vi "BC Next Frame Check.vi"(8 "error in (no error)":errorcluster, 11 "Bus Controller in":refnum<class "Bus Controller.lvclass">) -> (0 "error out":errorcluster, 3 "Bus Controller out":refnum<class "Bus Controller.lvclass">)   [LabVIEW 2020, in "Unit Tests.lvlib" / "Bus Controller.lvclass"]
uses:
  Bus Controller.lvclass
  Bus Controller.lvclass/Bus Controller.ctl
  Frames & Messages/TypeDefs/BC Condition Codes.ctl
  Frames & Messages/TypeDefs/BC Op Codes - Verbose.ctl
  <vilib>/addons/_JKI Toolkits/Caraya/classes/Assert/Assert True.vi
  Dependencies/FPGA Interface/FPGA Interface.lvclass
  <vilib>/addons/_JKI Toolkits/Caraya/classes/Test/Test.lvclass
  BCI-1553 API.lvlib
  <vilib>/addons/_JKI Toolkits/Caraya/classes/Assert/Assert.lvclass
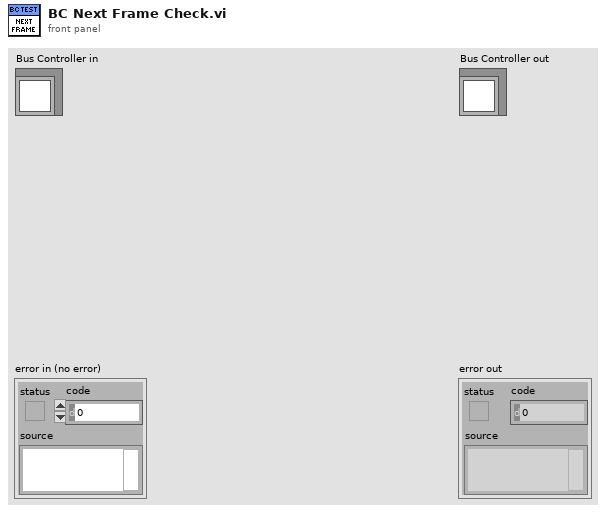
[diagram p1: front panel]
types:
  T1 = typedef "BCI-1553 API.lvlib/BC Op Codes - Verbose.ctl" = enum16{"EXECUTE MSG", "EXECUTE MSG GO", "JUMP", "CALL SUBROUTINE", "RETURN", "INTERRUPT REQUEST", "HALT", "DELAY", "WAIT FRAME TIMER = 0", "COMPARE FRAME TIMER", "COMPARE MSG TIMER", "LOAD TIME TAG CTR", "LOAD TIME TAG CTR HI", "LOAD FRAME TIMER", "START FRAME TIMER", "PUSH TIME TAG COUNT", "PUSH TIME TAG COUNT HI", "PUSH TIME TAG COUNT BOTH", "PUSH BLOCK STATUS WORD", "PUSH CURRENT VALUE", "PUSH INDIRECT", "WAIT EXT TRIGGER", "EXECUTE AND FLIP", "EXECUTE, FLIP, GO", "WRITE VALUE TO WMI", "WRITE VALUE TO MEM", "DECREMENT RAM, SKIP", "FLAG"}
  T2 = typedef "BCI-1553 API.lvlib/BC Condition Codes.ctl" = enum16{"GP0 == 1 || LT", "GP1 == 1 || NE", "GP2 == 1", "GP3 == 1", "GP4 == 1", "GP5 == 1", "GP6 == 1", "GP7 == 1", "NORESP", "FMTERR", "GOODBLOCK", "MSKSTATSET", "BADMSG", "1RETRY", "2RETRY", "ALWAYS"}
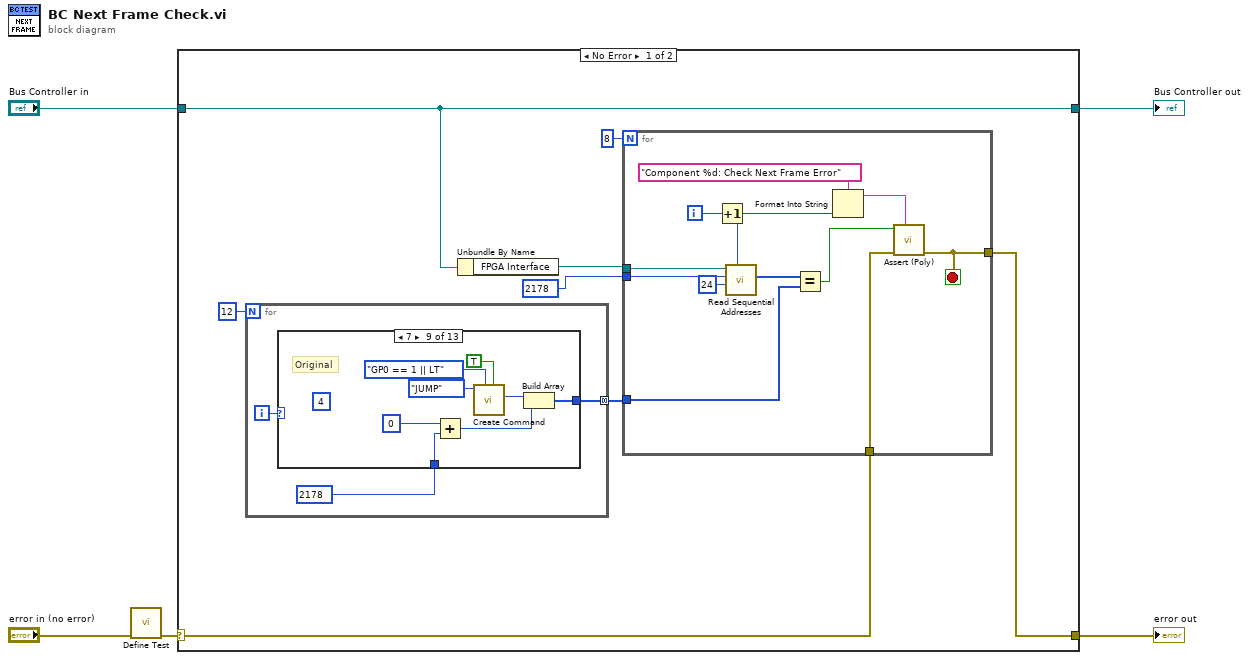
[diagram p0: block diagram]
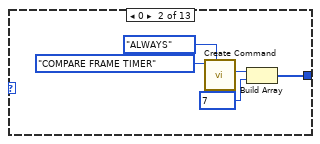
[diagram p3: hidden frame]
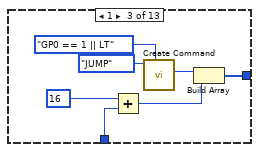
[diagram p4: hidden frame]
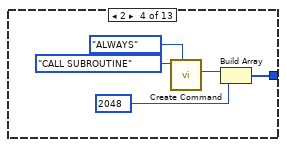
[diagram p5: hidden frame]
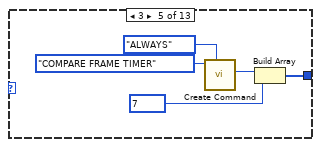
[diagram p6: hidden frame]
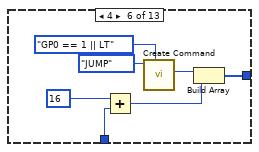
[diagram p7: hidden frame]
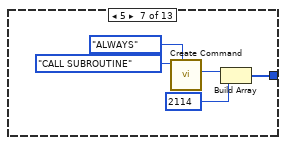
[diagram p8: hidden frame]
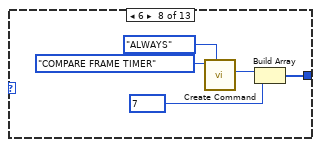
[diagram p9: hidden frame]
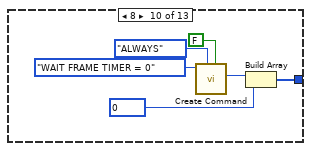
[diagram p10: hidden frame]
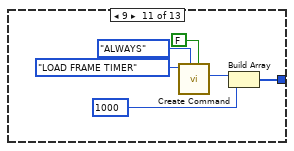
[diagram p11: hidden frame]
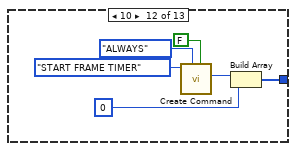
[diagram p12: hidden frame]
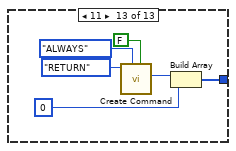
[diagram p13: hidden frame]
diagram:
  n1 = call <vilib>:"Define Test.vi"("error in (no error)"="error in (no error)") -> ("error out"=w1:errorcluster)  [unwired: 9 in, 1 out]
  n2 = case shown="No Error" w1 {
    selector: w1 -> [w8 w101]
    tunnel: [w7 w101] -> w5
    tunnel: [w11 w100] -> w3
    tunnel: "Bus Controller in" -> [w11 w100]
    frame No Error {
      n3 = for {
        N: 12 -> [_]
        tunnel: [w27] -> w12 mode=concatenating
        i -> [w28]
        n4 = case shown="7" w28 {
          tunnel: [_ w30 w37 w42 w47 w54 w59 w64 w72 w78 w84 w90 w96] -> w27
          tunnel: u16 2178 -> [_ _ w34 _ _ w51 _ _ w68 _ _ _ _]
          frame Default {
          }
          frame 0 {
            n5 = call "Create Command.vi"("Condition"=BC_Condition_Codes."ALWAYS", "Op Code"=BC_Op_Codes_-_Verbose."COMPARE FRAME TIMER") -> ("Instruction"=w31:u16)  [unwired: 8 in, 1 out]
            n6 = Build Array(w31, u16 7 ("element")) -> (w30:u16[])
          }
          frame 1 {
            n7 = Add(x=u16 16 ("element"), y=w34) -> (x+y=w36:u16)
            n8 = call "Create Command.vi"("Condition"=BC_Condition_Codes."GP0 == 1 || LT", "Op Code"=BC_Op_Codes_-_Verbose."JUMP") -> ("Instruction"=w38:u16)  [unwired: 8 in, 1 out]
            n9 = Build Array(w38, w36) -> (w37:u16[])
          }
          frame 2 {
            n10 = call "Create Command.vi"("Condition"=BC_Condition_Codes."ALWAYS", "Op Code"=BC_Op_Codes_-_Verbose."CALL SUBROUTINE") -> ("Instruction"=w43:u16)  [unwired: 8 in, 1 out]
            n11 = Build Array(w43, u16 2048) -> (w42:u16[])
          }
          frame 3 {
            n12 = call "Create Command.vi"("Condition"=BC_Condition_Codes."ALWAYS", "Op Code"=BC_Op_Codes_-_Verbose."COMPARE FRAME TIMER") -> ("Instruction"=w48:u16)  [unwired: 8 in, 1 out]
            n13 = Build Array(w48, u16 7) -> (w47:u16[])
          }
          frame 4 {
            n14 = Add(x=u16 16 ("element"), y=w51) -> (x+y=w52:u16)
            n15 = call "Create Command.vi"("Condition"=BC_Condition_Codes."GP0 == 1 || LT", "Op Code"=BC_Op_Codes_-_Verbose."JUMP") -> ("Instruction"=w55:u16)  [unwired: 8 in, 1 out]
            n16 = Build Array(w55, w52) -> (w54:u16[])
          }
          frame 5 {
            n17 = call "Create Command.vi"("Condition"=BC_Condition_Codes."ALWAYS", "Op Code"=BC_Op_Codes_-_Verbose."CALL SUBROUTINE") -> ("Instruction"=w60:u16)  [unwired: 8 in, 1 out]
            n18 = Build Array(w60, u16 2114) -> (w59:u16[])
          }
          frame 6 {
            n19 = call "Create Command.vi"("Condition"=BC_Condition_Codes."ALWAYS", "Op Code"=BC_Op_Codes_-_Verbose."COMPARE FRAME TIMER") -> ("Instruction"=w65:u16)  [unwired: 8 in, 1 out]
            n20 = Build Array(w65, u16 7) -> (w64:u16[])
          }
          frame 7 {
            (unwired) u16 4 ("element")
            # "Original"
            n21 = Add(x=u16 0 ("element"), y=w68) -> (x+y=w70:u16)
            n22 = call "Create Command.vi"("Invert Condition (F)"=TRUE, "Condition"=BC_Condition_Codes."GP0 == 1 || LT", "Op Code"=BC_Op_Codes_-_Verbose."JUMP") -> ("Instruction"=w73:u16)  [unwired: 7 in, 1 out]
            n23 = Build Array(w73, w70) -> (w72:u16[])
          }
          frame 8 {
            n24 = call "Create Command.vi"("Invert Condition (F)"=FALSE, "Condition"=BC_Condition_Codes."ALWAYS", "Op Code"=BC_Op_Codes_-_Verbose."WAIT FRAME TIMER = 0") -> ("Instruction"=w79:u16)  [unwired: 7 in, 1 out]
            n25 = Build Array(w79, u16 0) -> (w78:u16[])
          }
          frame 9 {
            n26 = call "Create Command.vi"("Invert Condition (F)"=FALSE, "Condition"=BC_Condition_Codes."ALWAYS", "Op Code"=BC_Op_Codes_-_Verbose."LOAD FRAME TIMER") -> ("Instruction"=w85:u16)  [unwired: 7 in, 1 out]
            n27 = Build Array(w85, u16 1000) -> (w84:u16[])
          }
          frame 10 {
            n28 = call "Create Command.vi"("Invert Condition (F)"=FALSE, "Condition"=BC_Condition_Codes."ALWAYS", "Op Code"=BC_Op_Codes_-_Verbose."START FRAME TIMER") -> ("Instruction"=w91:u16)  [unwired: 7 in, 1 out]
            n29 = Build Array(w91, u16 0) -> (w90:u16[])
          }
          frame 11 {
            n30 = call "Create Command.vi"("Invert Condition (F)"=FALSE, "Condition"=BC_Condition_Codes."ALWAYS", "Op Code"=BC_Op_Codes_-_Verbose."RETURN") -> ("Instruction"=w97:u16)  [unwired: 7 in, 1 out]
            n31 = Build Array(w97, u16 0) -> (w96:u16[])
          }
        }
      }
      n32 = Unbundle By Name(w11) -> ("FPGA Interface"=w10:refnum<class "FPGA Interface.lvclass">)
      n33 = for {
        N: 8 -> [_]
        tunnel: w10 -> [w25]
        tunnel: u16 2178 -> [w22]
        tunnel: [w16] -> w7
        tunnel: w12 -> [w18]
        tunnel: w8 -> [w14]
        i -> [w23]
        stop <- w16 stop-if-true
        n34 = Increment(x=w23) -> (x+1=w20:i32)
        n35 = call-dynamic "Read Sequential Addresses.vi"("Target IC (1-8)"=w20, "Addresses to Read"=u16 24, "Starting Address"=w22, "FPGA Interface in"=w25) -> ("Data"=w19:u16[])  [unwired: 6 in, 1 out]
        n36 = Equal?(x=w19, y=w18) -> (x = y?=w17:bool)
        n37 = Format Into String(format string="Component %d: Check Next Frame Error" ("custom report message (\"\")"), w20) -> (resulting string=w15:string)  [unwired: 2 in, 1 out]
        n38 = call-poly <vilib>:"Assert (Poly).vi"("Label"=w15, "error in (no error)"=w14, "True?"=w17) -> ("error out"=w16:errorcluster)  [unwired: 7 in, 1 out]
      }
    }
    frame Error {
    }
  }
  "error out" <- w5
  "Bus Controller out" <- w3
